vi "string_to_int_array.vi"(8 "error in (no error)":errorcluster, 10 "Ints":string) -> (0 "error out":errorcluster, 2 "Int array":i32[](array[numeric]))   [LabVIEW 2018, in "Inficon IC6.lvlib"]
doc: "Convert an IC6 response string representing a concetenated list of signed integers into an array of LabVIEW I32."
uses:
  <instrlib>/Inficon IC6/Inficon IC6.lvlib
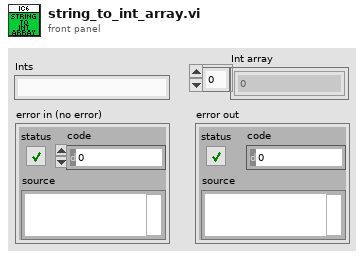
[diagram p1: front panel]
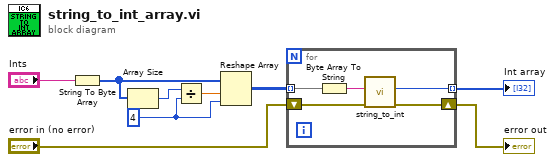
[diagram p0: block diagram]
diagram:
  w8 = 4 ("dimension size")
  n1 = String To Byte Array(string="Ints") -> (unsigned byte array=w1:u8[])
  n2 = Array Size(array=w1) -> (size(s)=w7:i32)
  n3 = Divide(x=w7, y=w8) -> (x/y=w6:dbl)
  n4 = Reshape Array(w1, w6, w8) -> (w5:u8[][])
  n5 = for {
    tunnel: [w13] -> w3 mode=indexing
    tunnel: w5 -> [w12] mode=indexing
    shift-right: [w11] -> w2
    shift-left: "error in (no error)" -> [w10]
    n6 = Byte Array To String(unsigned byte array=w12) -> (string=w14:string)
    n7 = call <instrlib>:"string_to_int.vi"("error in (no error)"=w10, "Int (string)"=w14) -> ("error out"=w11:errorcluster, "Int"=w13:i32)  [unwired: 8 in]
  }
  "Int array" <- w3
  "error out" <- w2
